vi "principal_app.vi"() -> ()   [LabVIEW 2013]
uses:
  subVI/bus to create file.ctl
  subVI/data simulation bus.ctl
  subVI/VoltElectrodo.ctl
  <vilib>/DAQmx/create/channels.llb/DAQmx Create Channel (AI-Voltage-Basic).vi
  <vilib>/addons/control/pid/pid.llb/PID Advanced (DBL).vi
  <vilib>/addons/System Identification/NI_SysID.lvlib
  <vilib>/addons/control/pid/NI_PID_pid.lvlib
panel:
  in  "PID gains":T1={"proportional gain (Kc)"=1.0, "integral time (Ti, min)"=0.01, "derivative time (Td, min)"=0.0} {"derivative time (Td, min)" format="%.3f"; "integral time (Ti, min)" format="%.3f"; "proportional gain (Kc)" format="%.3f"}
  in  "Nivel ref.":dbl
  in  "auto? (T)":bool
  out "v altura":dbl
  in  "Boolean":bool
  out "gasholdup":dbl(graph)
  out "gas holdup":dbl
  out "Flotation column":dbl(slide)
  out "Altura capa de espuma":dbl(graph)
  in  "Procesar datos\nen Matlab":bool
  in  "Record":bool
  out "output cluster":cluster{"pulp flow":dbl, "gang flow":dbl}(graph)
  in  "Emergency  \nopen/close \nvalve":bool
  out "Max non floated Flow":bool
  in  "STOP":bool
  out "right corner pipe 2":bool
  out "Max Air Flow":bool
  out "Water Flow":bool
  out "Max Pulp Flow":bool
  in  "Power\nPumps":bool
  in  "Water ref":i32 min=0 max=4003
  out "MFC Water":bool
  out "Water pump":bool
  out "water pipe":bool
  out "Air compressor":bool
  in  "Air reference":u16 max=100 step=1
  out "MFC Air":bool
  out "air pipe":bool
  in  "Gang ref":u16 max=1600 step=1
  out "MFC Gang":bool
  out "gang pipe":bool
  in  "Pulp ref":u16 max=1693
  out "MFC Pulp":bool
  out "pulp pipe":bool
  out "Pulp pump":bool
  out "Air flow":i16(graph)
  # "Flow : (200) [ml/min]"
  # "Flow : (0 - 1693) [ml/min]"
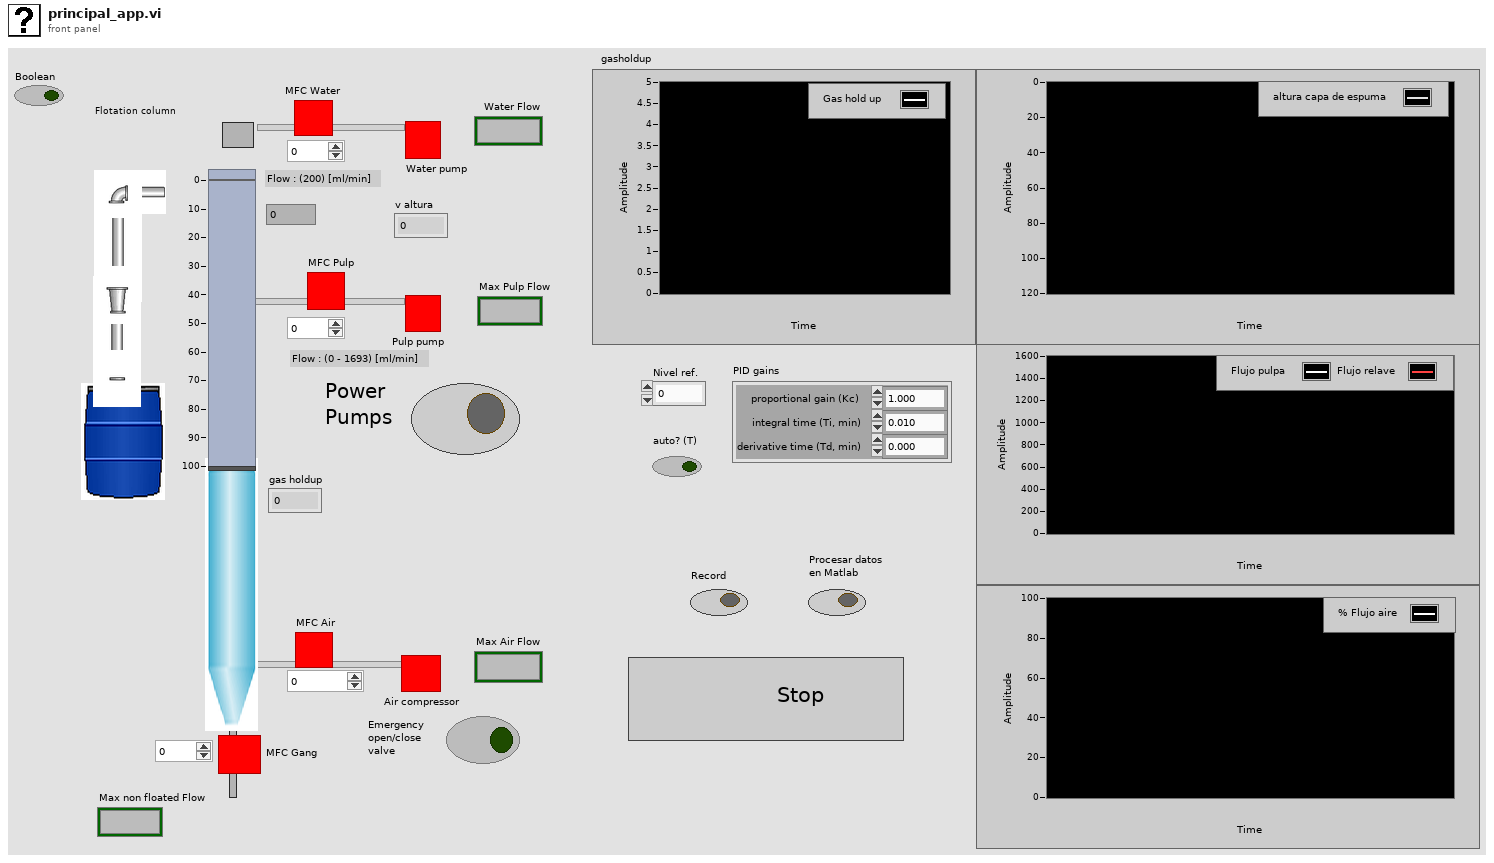
[diagram p1: front panel]
types:
  T1 = cluster{"proportional gain (Kc)":dbl, "integral time (Ti, min)":dbl, "derivative time (Td, min)":dbl}
  T2 = typedef "bus to create file.ctl" = cluster{"data simulation":T3, "Time":dbl, "volt":T4}
  T3 = typedef "data simulation bus.ctl" = cluster{"Flujo pulpa ":dbl, "Flujo agua lavado":dbl, "Flujo aire":dbl, "Flujo relave":dbl, "Altura capa de espuma":dbl, "Gas holdup":dbl, "% apertura valvula aire":dbl, "ref pulp":dbl}
  T4 = typedef "VoltElectrodo.ctl" = cluster{"V1":dbl, "V2":dbl, "V3":dbl, "V4":dbl, "V5":dbl, "V6":dbl, "V7":dbl, "V8":dbl}
  T5 = typedef "medidas.ctl" = cluster{"Water Flow":bool, "encendido electrobomba":bool, "pulp flow":dbl, "water flow":dbl, "max pulp flow":bool, "Medicion Flujometro":u16, "max non floated flow ":bool, "gang flow":dbl}
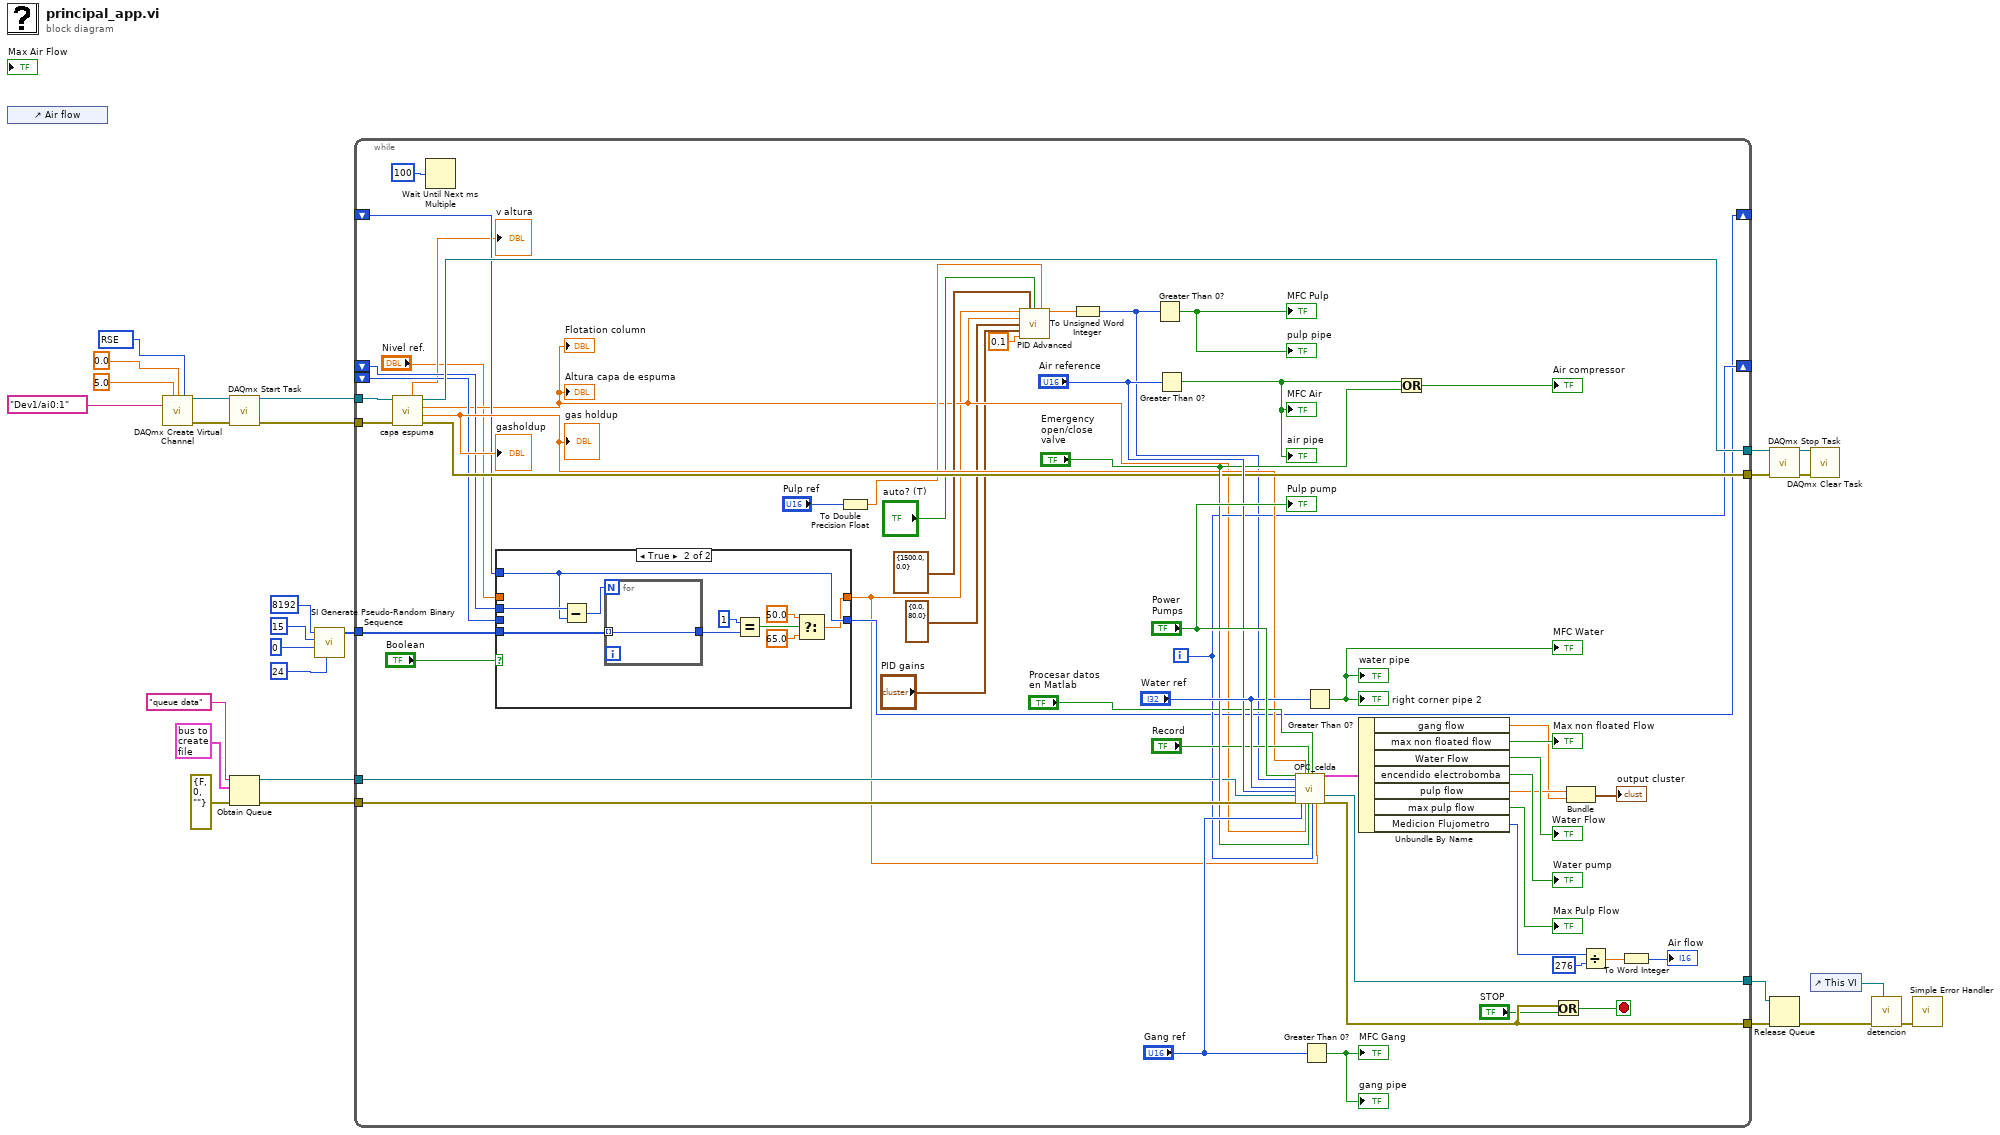
[diagram p0: block diagram]
diagram:
  w11 = 10083 items=["default"=-1, "RSE"=10083, "NRSE"=10078, "Differential"=10106, "Pseudodifferential"=12529] ("input terminal configuration")
  n1 = control-ref of="Air flow"() -> ()  [unwired: 1 out]
  n2 = call-poly <vilib>:"DAQmx Create Virtual Channel.vi"("maximum value"=5.0, "minimum value"=0.0, "input terminal configuration"=w11, "physical channels"=tag "Dev1/ai0:1") -> ("task out"=w20:refnum<k21>, "error out"=w14:errorcluster)  [unwired: 10 in]
  n3 = call <vilib>:"DAQmx Start Task.vi"("task/channels in"=w20, "error in"=w14) -> ("task out"=w19:refnum<k21>, "error out"=w9:errorcluster)  [unwired: 12 in]
  n4 = Obtain Queue(name (unnamed)="queue data", element data type=T2 {"data simulation"={"Flujo pulpa "=0.0, "Flujo agua lavado"=0.0, "Flujo aire"=0.0, "Flujo relave"=0.0, "Altura capa de espuma"=0.0, "Gas holdup"=0.0, "% apertura valvula aire"=0.0, "ref pulp"=0.0}, "Time"=0.0, "volt"={"V1"=0.0, "V2"=0.0, "V3"=0.0, "V4"=0.0, "V5"=0.0, "V6"=0.0, "V7"=0.0, "V8"=0.0}}, error in (no error)=errorcluster {"status"=FALSE, "code"=0, "source"=""}) -> (queue out=w25:refnum<queue>, error out=w21:errorcluster)  [unwired: 2 in, 1 out]
  n5 = call <vilib>:"SI Generate Pseudo-Random Binary Sequence.vi"("upsampling factor"=24, "seed"=i64 0, "polynomial order"=15, "samples"=i64 8192) -> ("PRBS"=w5:u8[])  [unwired: 7 in]
  n6 = while {
    tunnel: [w72] -> w23
    tunnel: w21 -> [w74]
    tunnel: [w61] -> w24
    tunnel: w25 -> [w60]
    tunnel: w19 -> [w58]
    tunnel: w9 -> [w57]
    tunnel: [w56] -> w18
    tunnel: [w55] -> w15
    tunnel: w5 -> [w51]
    shift-right: [w50] -> _
    shift-left: _ -> [w49]
    shift-left: _ -> [w47]
    shift-right: [w48] -> _
    shift-left: _ -> [w46]
    i -> [w50]
    stop <- w73 stop-if-true
    n7 = call "capa espuma.vi"("error in (no error)"=w57, "Refnum in"=w58) -> ("error out"=w56:errorcluster, "gas holdup"=w52:dbl, "Flotation column"=w33:dbl, "Refnum out"=w55:refnum<k21>, "element"=→"v altura":dbl)  [unwired: 5 in]
    "Flotation column" <- w33
    "Altura capa de espuma" <- w33
    "gas holdup" <- w52
    "gasholdup" <- w52
    n8 = Wait Until Next ms Multiple(millisecond multiple=u32 100) -> ()  [unwired: 1 out]
    n9 = case shown="True" "Boolean" {
      tunnel: w51 -> [_ w95]
      tunnel: w49 -> [_ w94]
      tunnel: [w85 w93] -> w48
      tunnel: w47 -> [w85 _]
      tunnel: w46 -> [_ w93]
      tunnel: [w84 w86] -> w28
      tunnel: "Nivel ref." -> [w84 _]
      frame False {
      }
      frame True {
        n10 = Subtract(x=w94, y=w93) -> (x-y=w92:i32)
        n11 = for {
          N: w92 -> [_]
          tunnel: w95 -> [w96] mode=indexing
          tunnel: [w96] -> w91
        }
        n12 = Equal?(x=u8 1, y=w91) -> (x = y?=w89:bool)
        n13 = Select(t=50.0, s=w89, f=65.0) -> (s? t:f=w86:dbl)
      }
    }
    n14 = To Double Precision Float(number="Pulp ref") -> (double precision float=w34:dbl)
    n15 = call-poly <vilib>:"PID Advanced.vi"("setpoint"=w28, "output range"=cluster{"output high":dbl, "output low":dbl} {"output high"=1500.0, "output low"=0.0}, "auto? (T)"="auto? (T)", "manual control"=w34, "process variable"=w33, "setpoint range"=cluster{"setpoint high":dbl, "setpoint low":dbl} {"setpoint high"=0.0, "setpoint low"=80.0}, "PID gains"="PID gains", "dt (s)"=0.1) -> ("output"=w38:dbl)  [unwired: 6 in, 1 out]
    n16 = To Unsigned Word Integer(number=w38) -> (unsigned 16bit integer=w37:u16)
    n17 = Greater Than 0?(x=w37) -> (x > 0?=→"MFC Pulp" →"pulp pipe":bool)
    n18 = Greater Than 0?(x="Air reference") -> (x > 0?=w67:bool)
    "MFC Air" <- w67
    "air pipe" <- w67
    n19 = call "OPC_celda.vi"("power"="Power\nPumps", "Pulp ref"=w37, "water ref"="Water ref", "Setpoint Flujometro"="Air reference", "queue"=w60, "error in (no error)"=w74, "Gang ref"="Gang ref", "Gas holdup"=w52, "Altura capa de espuma"=w33, "Record"="Record", "emergency  \nopen/close \nvalve"="Emergency  \nopen/close \nvalve", "Procesar datos\nen Matlab"="Procesar datos\nen Matlab", "iteration"=w50, "ref pulp"=w28) -> ("output cluster"=w79:T5, "queue out"=w61:refnum<queue>, "error out"=w72:errorcluster)  [unwired: 11 in]
    n20 = Greater Than 0?(x="Gang ref") -> (x > 0?=→"gang pipe" →"MFC Gang":bool)
    n21 = Greater Than 0?(x="Water ref") -> (x > 0?=→"MFC Water" →"water pipe" →"right corner pipe 2":bool)
    n22 = Unbundle By Name(w79) -> ("gang flow"=w62:dbl, "max non floated flow"=→"Max non floated Flow":bool, "Water Flow"=→"Water Flow":bool, "encendido electrobomba"=→"Water pump":bool, "pulp flow"=w64:dbl, "max pulp flow"=→"Max Pulp Flow":bool, "Medicion Flujometro"=w45:u16)
    n23 = Or(x=w67, y="Emergency  \nopen/close \nvalve") -> (x .or. y?=→"Air compressor":bool)
    n24 = Or(x=w72, y="STOP") -> (x .or. y?=w73:bool)
    n25 = Bundle("pulp flow"=w64, "gang flow"=w62) -> (→"output cluster":cluster{"pulp flow":dbl, "gang flow":dbl})  [unwired: 1 in]
    n26 = Divide(x=w45, y=u16 276) -> (x/y=w43:dbl)
    n27 = To Word Integer(number=w43) -> (16bit integer=→"Air flow":i16)
    "Pulp pump" <- "Power\nPumps"
  }
  n28 = call <vilib>:"DAQmx Stop Task.vi"("task/channels in"=w15, "error in"=w18) -> ("task out"=w16:refnum<k21>, "error out"=w17:errorcluster)  [unwired: 12 in]
  n29 = Release Queue(queue=w24, error in (no error)=w23) -> (error out=w22:errorcluster)  [unwired: 1 in, 2 out]
  n30 = call <vilib>:"DAQmx Clear Task.vi"("task in"=w16, "error in"=w17) -> ()  [unwired: 13 in, 1 out]
  n31 = control-ref of="This VI"() -> (w27:refnum<vi>)
  n32 = call "detencion.vi"("This VI"=w27, "error in (no error)"=w22) -> ("error out"=w26:errorcluster)  [unwired: 9 in]
  n33 = call <vilib>:"Simple Error Handler.vi"("error in (no error)"=w26) -> ()  [unwired: 4 in, 5 out]
